vi "Sleeping.vi"() -> ()   [LabVIEW 2025]
uses:
  <vilib>/Instr/_visa.llb/VISA Configure Serial Port (Instr).vi
panel:
  in  "session in":refnum<k35>
  out "return value":string
  out "Risk":string="Risk"
  out "read buffer":string
  out "?":string
  in  "stop":bool
  out "Heart Rate":dbl
  out "Body_temp":dbl
  out "Humidity":dbl
  out "Room_temp":dbl
  out "Sp02":dbl
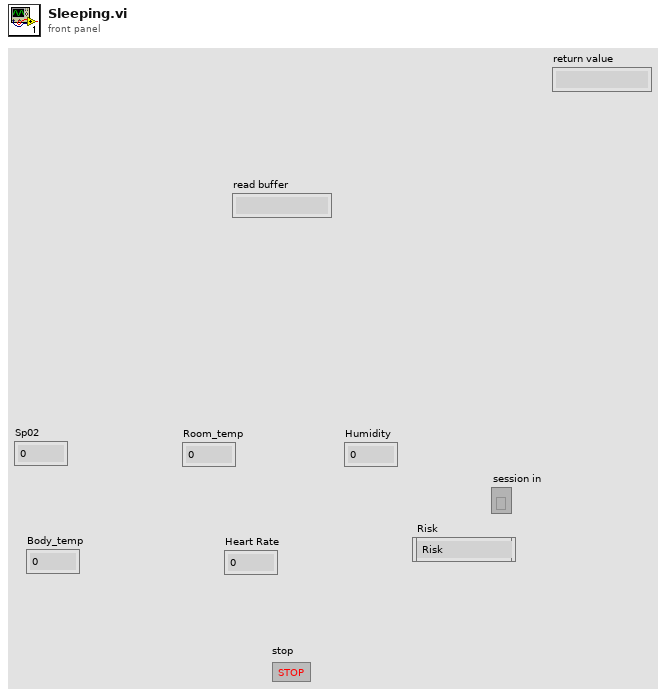
[diagram p1: front panel]
types:
  T1 = enum16{"open", "replace", "create", "open or create", "replace or create", "replace or create with confirmation"}
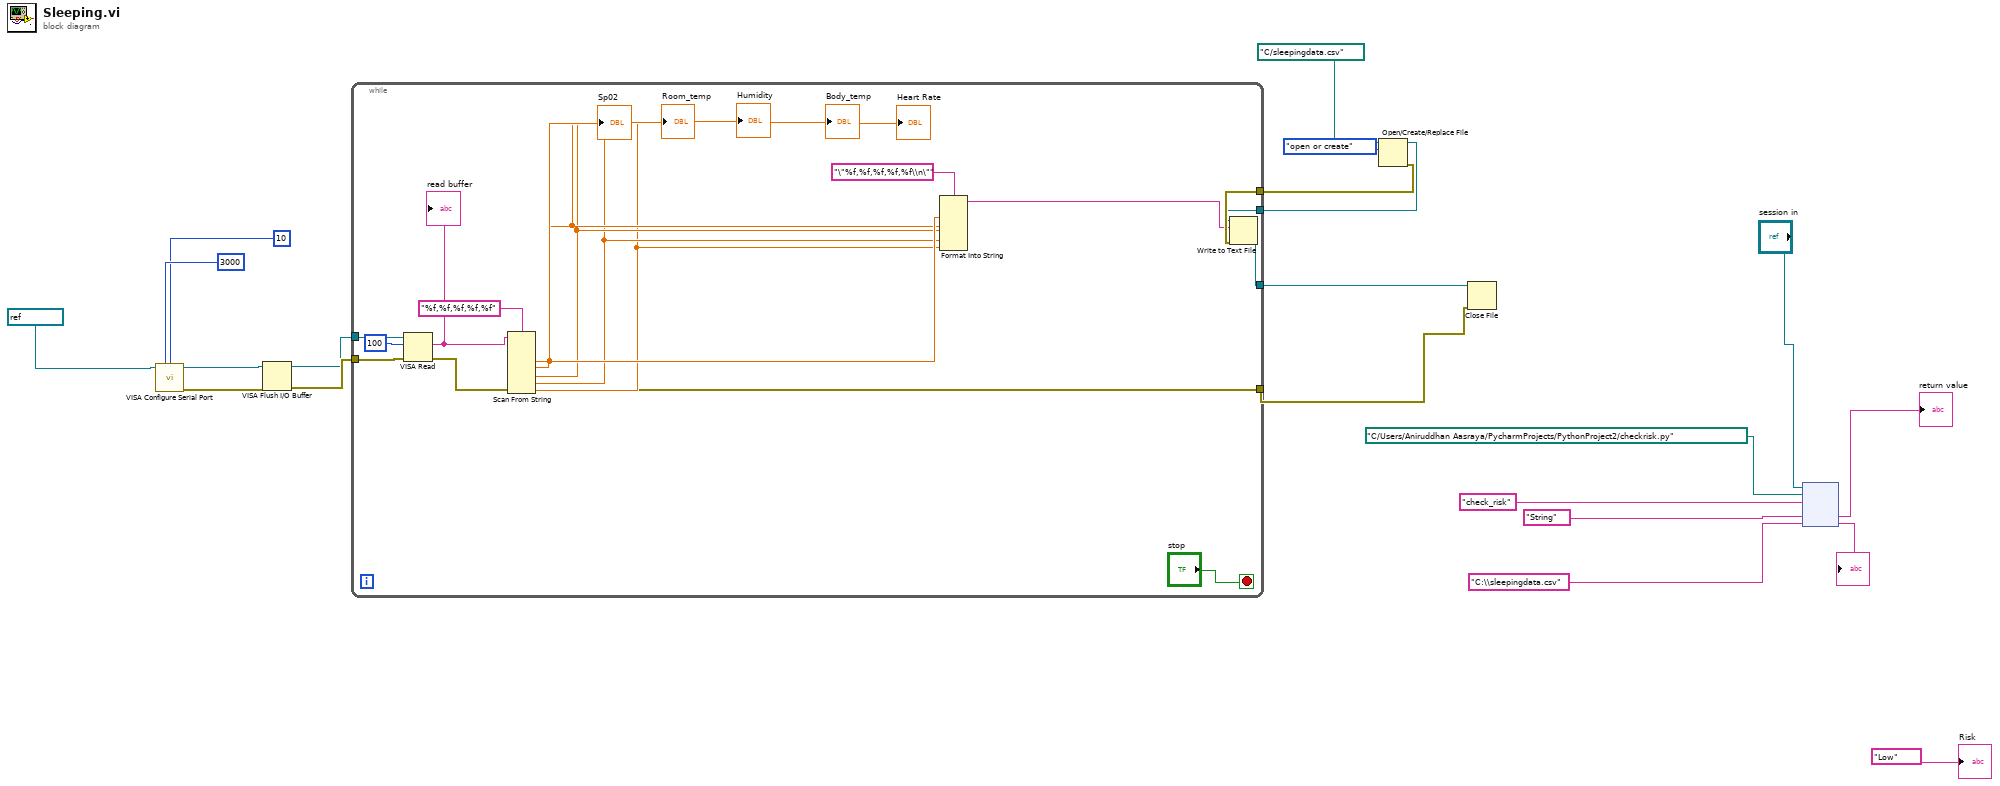
[diagram p0: block diagram]
diagram:
  n1 = call-poly "VISA Configure Serial Port"("VISA resource name"=refnum<visa-resource-name> "COM4", "timeout (10sec)"=u32 3000, "termination char\n(0xA = '\\n' = LF)"=u8 10 ("termination char\n(0xA = '\\n' = LF)")) -> ("VISA resource name out"=w4:refnum<visa-resource-name>, "error out"=w3:errorcluster)  [unwired: 11 in]
  n2 = VISA Flush I/O Buffer(VISA resource name=w4, error in (no error)=w3) -> (VISA resource name out=w1:refnum<visa-resource-name>, error out=w2:errorcluster)  [unwired: 1 in]
  n3 = Open/Create/Replace File(file path (use dialog)=path "C:/sleepingdata.csv", operation (0:open)=T1."open or create") -> (refnum out=w17:refnum<file>, error out=w18:errorcluster)  [unwired: 4 in, 1 out]
  n4 = while {
    tunnel: w1 -> [w36]
    tunnel: w2 -> [w35]
    tunnel: [w26] -> w8
    tunnel: w18 -> [w25]
    tunnel: w17 -> [w23]
    tunnel: [w22] -> w16
    stop <- "stop" stop-if-true
    n5 = VISA Read(VISA resource name=w36, byte count=u32 100, error in (no error)=w35) -> (read buffer=w34:string, error out=w26:errorcluster)  [unwired: 2 out]
    "read buffer" <- w34
    n6 = Scan From String(format string="%f,%f,%f,%f,%f", input string=w34) -> (output 1=w32:dbl, output 2=w31:dbl, output 3=w30:dbl, output 4=w29:dbl, output 5=w28:dbl)  [unwired: 7 in, 3 out]
    "Sp02" <- w32
    "Room_temp" <- w31
    "Humidity" <- w30
    "Body_temp" <- w29
    "Heart Rate" <- w28
    n7 = Format Into String(format string="\"%f,%f,%f,%f,%f\\n\"", w32, w31, w30, w29, w28) -> (resulting string=w24:string)  [unwired: 2 in, 1 out]
    n8 = Write to Text File(file (use dialog)=w23, text=w24, error in=w25) -> (refnum out=w22:refnum<file>)  [unwired: 1 in, 2 out]
  }
  n9 = Close File(refnum=w16, error in=w8) -> ()  [unwired: 2 out]
  n10 = node("session in", path "C:/Users/Aniruddhan Aasraya/PycharmProjects/PythonProject2/checkrisk.py" ("module path"), "check_risk" ("function name"), "String", "C:\\sleepingdata.csv") -> (→"return value":string, →"?":string)  [unwired: 1 in, 4 out]
  "Risk" <- "Low"
